vi "Is New Trial - graph loop.vi"(1 "Position data":dbl, 2 "Minimum value drop":dbl=-50.0) -> (0 "Boolean":bool)   [LabVIEW 2017]
panel:
  out "count 1":dbl
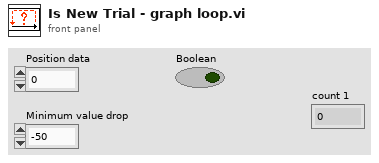
[diagram p1: front panel]
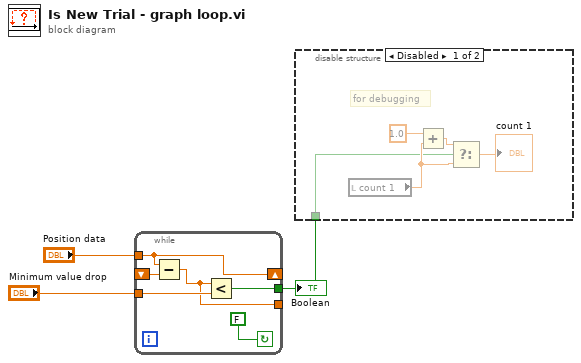
[diagram p0: block diagram]
diagram:
  n1 = while {
    shift-left: _ -> [w7]
    shift-right: [w8] -> _
    tunnel: "Position data" -> [w8]
    tunnel: "Minimum value drop" -> [w6]
    tunnel: [w5] -> w1
    tunnel: [w4] -> _
    stop <- FALSE continue-if-true
    n2 = Subtract(x=w8, y=w7) -> (x-y=w4:dbl)
    n3 = Less?(x=w4, y=w6) -> (x < y?=w5:bool)
  }
  "Boolean" <- w1
  n4 = disable-structure shown="Disabled" {
    disable-tunnel: w1 -> [w10 _]
    frame Disabled {
      # "for debugging"
      n5 = local read "count 1"() -> (w13:dbl)
      n6 = Add(x=1.0, y=w13) -> (x+y=w12:dbl)
      n7 = Select(t=w12, s=w10, f=w13) -> (s? t:f=→"count 1":dbl)
    }
    frame Enabled {
    }
  }
